vi "Acquire Maze.vi"() -> ()   [LabVIEW 2012]
uses:
  <vilib>/vision/NI_Vision_Development_Module.lvlib
panel:
  in  "View (%)":sgl=100.0 min=0 max=100
  in  "Crop Point":i32=60 min=0 max=160 step=1
  out "Reduced Resolution":T1(plugin-control)
  out "Frame Rate":dbl
  out "Raw Feed":T1(plugin-control)
  in  "Stop (F)":bool
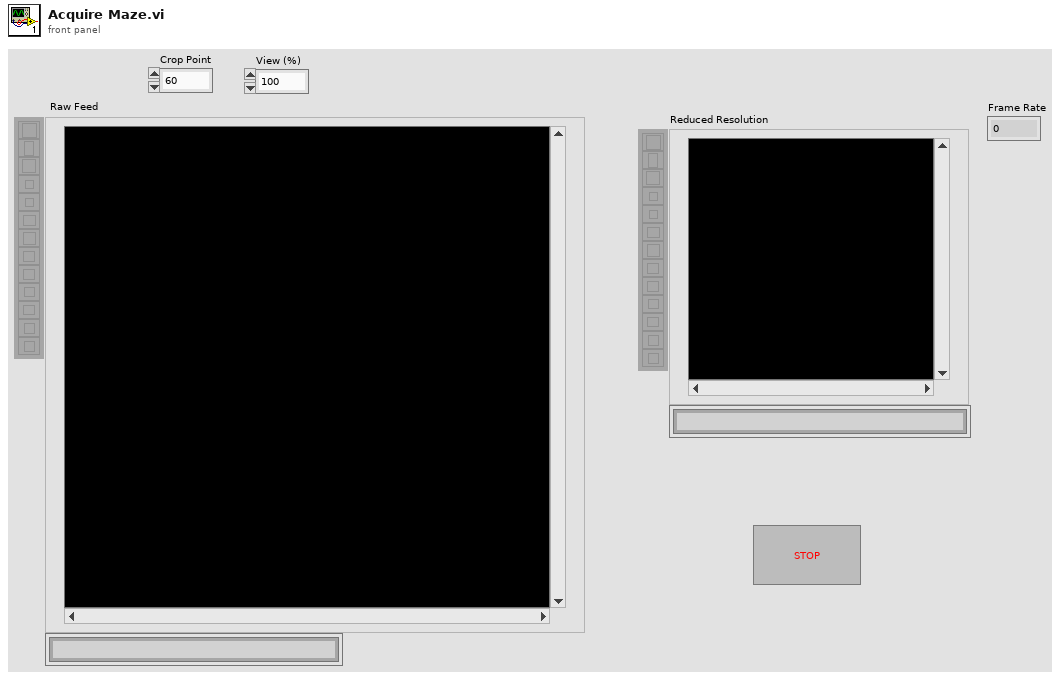
[diagram p1: front panel]
types:
  T1 = typedef "IMAQ Image.ctl" = refnum<image>
  T2 = typedef "Image Type" = u32
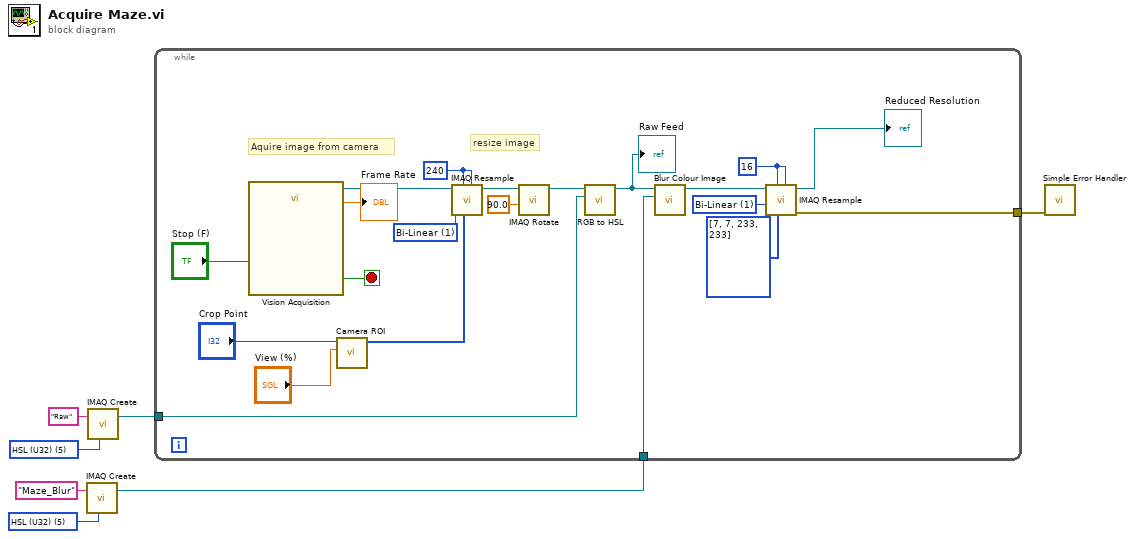
[diagram p0: block diagram]
diagram:
  w3 = T2 5 items=["Grayscale (U8)", "Grayscale (I16)", "Grayscale (SGL)", "Complex (CSG)", "RGB (U32)", "HSL (U32)", "RGB (U64)", "Grayscale (U16)"] ("Image Type")
  w6 = T2 5 items=["Grayscale (U8)", "Grayscale (I16)", "Grayscale (SGL)", "Complex (CSG)", "RGB (U32)", "HSL (U32)", "RGB (U64)", "Grayscale (U16)"] ("Image Type")
  n1 = call "IMAQ Create"("Image Name"="Maze_Blur", "Image Type"=w6) -> ("New Image"=w5:T1)  [unwired: 3 in, 1 out]
  n2 = call "IMAQ Create"("Image Name"="Raw", "Image Type"=w3) -> ("New Image"=w1:T1)  [unwired: 3 in, 1 out]
  n3 = while {
    tunnel: [w21] -> w7
    tunnel: w5 -> [w19]
    tunnel: w1 -> [w18]
    stop <- w27 stop-if-true
    w11 = 240 ("Y Resolution")
    w12 = u32 1 items=["Zero Order", "Bi-Linear", "Quadratic", "Cubic Spline"] ("Interpolation Type")
    w25 = 16 ("Y Resolution")
    w26 = u32 1 items=["Zero Order", "Bi-Linear", "Quadratic", "Cubic Spline"] ("Interpolation Type")
    # "resize image"
    # "Aquire image from camera"
    n4 = call "Vision Acquisition"("Stop (F)"="Stop (F)") -> ("Image Out"=w10:T1, "Frame Rate"=→"Frame Rate":dbl, "Stopped"=w27:bool)  [unwired: 23 in, 1 out]
    n5 = call "Camera ROI.vi"("View (%)"="View (%)", "Crop Point"="Crop Point") -> ("Camera ROI"=w15:i32[])  [unwired: 9 in]
    n6 = call "IMAQ Resample"("X Resolution"=w11, "Optional Rectangle"=w15, "Y Resolution"=w11, "Interpolation Type"=w12, "Image Src"=w10) -> ("Image Dst Out"=w8:T1)  [unwired: 5 in, 1 out]
    n7 = call "IMAQ Rotate"("Angle (degrees)"=sgl 90.0, "Image Src"=w8) -> ("Image Dst Out"=w20:T1)  [unwired: 8 in, 1 out]
    n8 = call "RGB to HSL.vi"("Destination (HSL)"=w18, "Image (RGB)"=w20) -> ("Image Out (HSL)"=w17:T1)  [unwired: 9 in]
    "Raw Feed" <- w17
    n9 = call "Blur Colour Image.vi"("Image Dest"=w19, "Image Src"=w17) -> ("Image Dest Out"=w23:T1)  [unwired: 9 in]
    n10 = call "IMAQ Resample"("X Resolution"=w25, "Optional Rectangle"=i32[] [7, 7, 233, 233], "Y Resolution"=w25, "Interpolation Type"=w26, "Image Src"=w23) -> ("error out"=w21:errorcluster, "Image Dst Out"=→"Reduced Resolution":T1)  [unwired: 5 in]
  }
  n11 = call <vilib>:"Simple Error Handler.vi"("error in (no error)"=w7) -> ()  [unwired: 1 in, 8 out]
